vi "imageObjectFind.vi"() -> ()   [LabVIEW 2011, in "run.lvlib"]
uses:
  run.lvlib
panel:
  out "element":T1
  in  "stop":bool
  in  "Rectangle":T2={"Left"=488, "Top"=341, "Right"=696, "Bottom"=565, "Rotation"=0.0} {"Rotation" format="%.2f"; "Left" scale=0.0..1024.0; "Right" scale=0.0..1024.0}
  out "Image":T3(plugin-control)
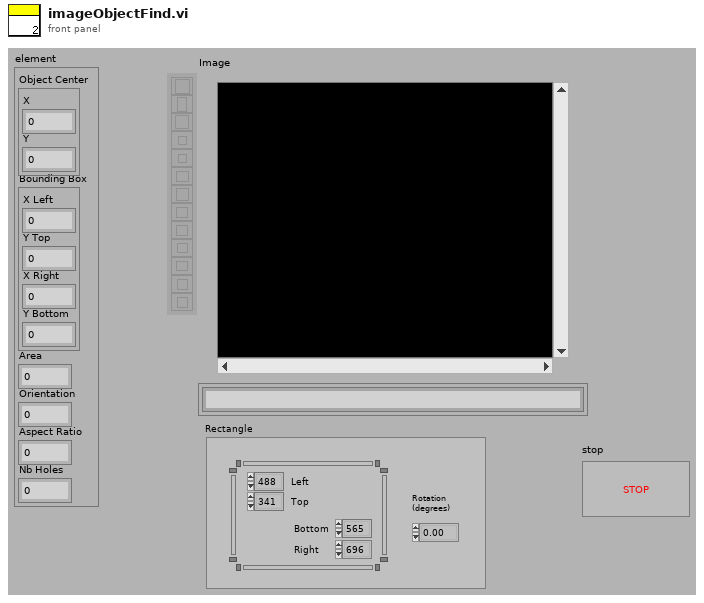
[diagram p1: front panel]
types:
  T1 = cluster{"Object Center":cluster{"X":sgl, "Y":sgl}, "Bounding Box":cluster{"X Left":i32, "Y Top":i32, "X Right":i32, "Y Bottom":i32}, "Area":sgl, "Orientation":sgl, "Aspect Ratio":sgl, "Nb Holes":i32}
  T2 = typedef "IMAQ Rectangle" = cluster{"Left":i32, "Top":i32, "Right":i32, "Bottom":i32, "Rotation":dbl}
  T3 = typedef "IMAQ Image.ctl" = refnum<image>
  T4 = cluster{"Left":i32, "Top":i32, "Right":i32, "Bottom":i32}
  T5 = typedef "Image Type" = u32
  T6 = cluster{"Objects":u16, "Threshold":i32, "Reject Border":bool, "Fill Holes":bool, "Min Object Size":bool, "Min Size":i32, "Max Object Size":bool, "Max Size":i32, "Show Search Area":bool, "Show Center":bool, "Show Bounding Box":bool}
  T7 = cluster{"Object Center":cluster{"X":sgl, "Y":sgl}, "Bounding Box":cluster{"X Left":i32, "Y Top":i32, "X Right":i32, "Y Bottom":i32}, "Area":sgl, "Orientation":sgl, "Aspect Ratio":sgl, "Nb Holes":i32}[]
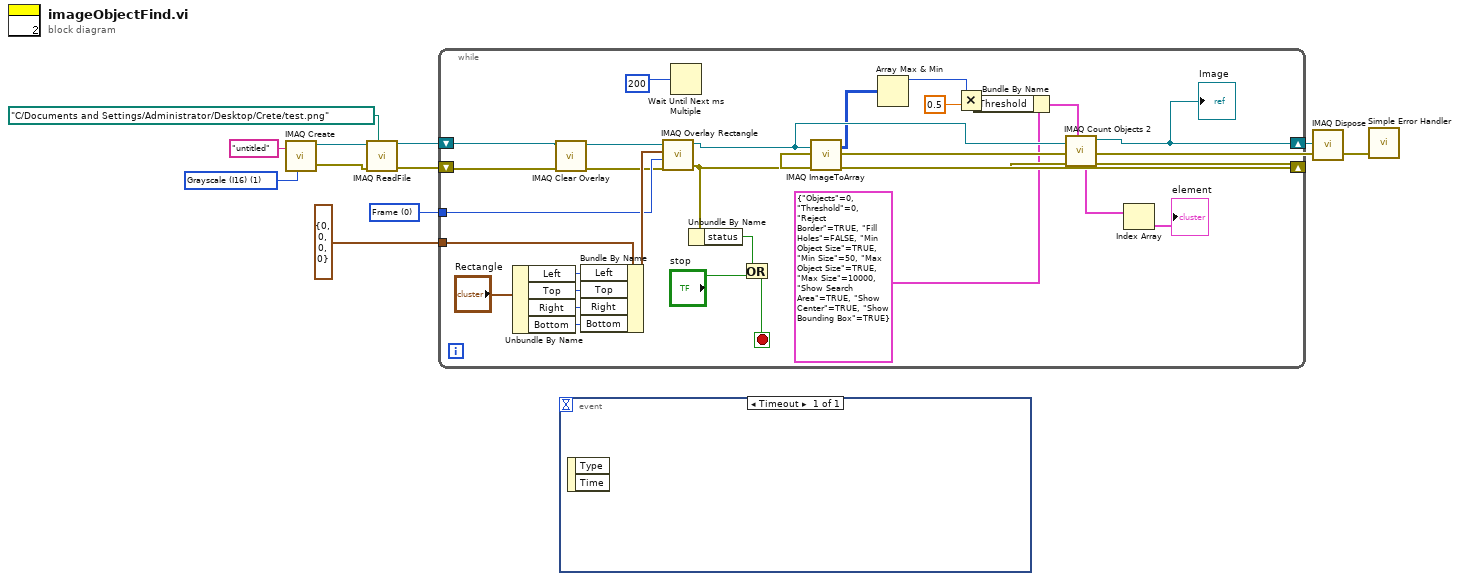
[diagram p0: block diagram]
diagram:
  w4 = u32 0 items=["Frame", "Fill", "Highlight"] ("Drawing Mode (Frame)")
  w11 = T5 1 items=["Grayscale (U8)", "Grayscale (I16)", "Grayscale (SGL)", "Complex (CSG)", "RGB (U32)", "HSL (U32)", "RGB (U64)", "Grayscale (U16)"] ("Image Type")
  n1 = call "IMAQ Create"("Image Name"="untitled", "Image Type"=w11) -> ("New Image"=w10:T3, "error out"=w9:errorcluster)  [unwired: 3 in]
  n2 = call "IMAQ ReadFile"("File Path"=path "C:/Documents and Settings/Administrator/Desktop/Crete/test.png", "error in (no error)"=w9, "Image"=w10) -> ("error out"=w6:errorcluster, "Image Out"=w7:T3)  [unwired: 4 in, 3 out]
  n3 = while {
    shift-right: [w13] -> w3
    shift-left: w7 -> [w29]
    shift-right: [w16] -> w2
    shift-left: w6 -> [w26]
    tunnel: T4 {"Left"=0, "Top"=0, "Right"=0, "Bottom"=0} ("Rectangle 2") -> [w41]
    tunnel: w4 -> [w34]
    stop <- w31 stop-if-true
    n4 = Unbundle By Name("Rectangle") -> ("Left"=w39:i32, "Top"=w36:i32, "Right"=w37:i32, "Bottom"=w38:i32)
    n5 = call "IMAQ Clear Overlay"("error in (no error)"=w26, "Image"=w29) -> ("error out"=w27:errorcluster, "Image Out"=w28:T3)  [unwired: 8 in]
    n6 = Bundle By Name(cluster=w41, "Left"=w39, "Top"=w36, "Right"=w37, "Bottom"=w38) -> (w35:T4)
    n7 = call "IMAQ Overlay Rectangle"("error in (no error)"=w27, "Drawing Mode (Frame)"=w34, "Rectangle"=w35, "Image"=w28) -> ("error out"=w25:errorcluster, "Image Out"=w23:T3)  [unwired: 6 in]
    n8 = Wait Until Next ms Multiple(millisecond multiple=200) -> ()  [unwired: 1 out]
    n9 = Unbundle By Name(w25) -> ("status"=w33:bool)
    n10 = Or(x=w33, y="stop") -> (x .or. y?=w31:bool)
    n11 = call "IMAQ ImageToArray"("error in (no error)"=w25, "Image"=w23) -> ("error out"=w24:errorcluster, "Image Pixels (I16)"=w21:i16[][])  [unwired: 2 in, 3 out]
    n12 = Array Max & Min(array=w21) -> (max value=w20:i16)  [unwired: 3 out]
    n13 = Multiply(x=w20, y=0.5) -> (x*y=w19:dbl)
    n14 = Bundle By Name(cluster=T6 {"Objects"=0, "Threshold"=0, "Reject Border"=TRUE, "Fill Holes"=FALSE, "Min Object Size"=TRUE, "Min Size"=50, "Max Object Size"=TRUE, "Max Size"=10000, "Show Search Area"=TRUE, "Show Center"=TRUE, "Show Bounding Box"=TRUE} ("Settings"), "Threshold"=w19) -> (w17:T6)
    n15 = call "IMAQ Count Objects 2"("Settings"=w17, "error in (no error)"=w24, "Image"=w23) -> ("error out"=w16:errorcluster, "Image Out"=w13:T3, "Objects"=w15:T7)  [unwired: 4 in, 2 out]
    "Image" <- w13
    n16 = Index Array(array=w15) -> (element=→"element":T1)  [unwired: 1 in]
  }
  n17 = event shown="[0] Timeout" {
    selector: _ -> [_]
    dyn-events: _ -> [_]
    timeout: _ -> [_]
    event Timeout {
      n18 = event-data() -> ()  [unwired: 1 in, 2 out]
    }
  }
  n19 = call "IMAQ Dispose"("Image"=w3, "error in (no error)"=w2) -> ("error out"=w1:errorcluster)  [unwired: 4 in]
  n20 = call <vilib>:"Simple Error Handler.vi"("error in (no error)"=w1) -> ()  [unwired: 4 in, 5 out]
